vi "Release.vi"(8 "error in (no error)":errorcluster, 11 "Transporter in":refnum<class "Transporter.lvclass">) -> (0 "error out":errorcluster)   [LabVIEW 2021, in "Msn Trasnsportation Library 1.lvlib" / "Transporter.lvclass"]
uses:
  Transporter.lvclass
  Transporter.lvclass/Transporter.ctl
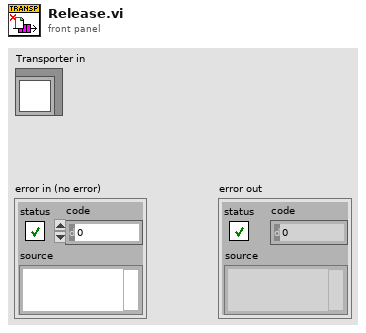
[diagram p1: front panel]
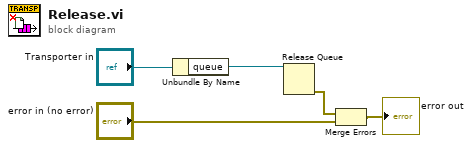
[diagram p0: block diagram]
diagram:
  n1 = Unbundle By Name("Transporter in") -> ("queue"=w4:refnum<queue>)
  n2 = Release Queue(queue=w4) -> (error out=w3:errorcluster)  [unwired: 2 in, 2 out]
  n3 = Merge Errors(w3, "error in (no error)") -> (→"error out":errorcluster)
